vi "Set External Result Ref.vi"(10 "External Result Ref":string, 11 "Test Run Result in":refnum<class "Test Run Result.lvclass">) -> (3 "Test Run Result out":refnum<class "Test Run Result.lvclass">)   [LabVIEW 2026, in "Test Run Result.lvclass"]
uses:
  Test Run Result.lvclass
  Test Run Result.lvclass/Test Run Result.ctl
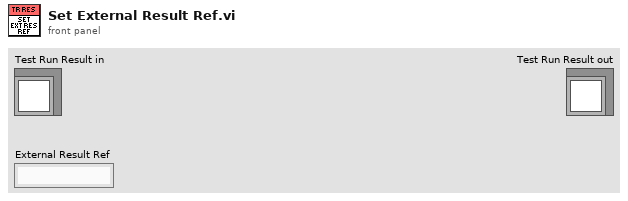
[diagram p1: front panel]
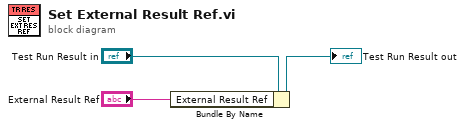
[diagram p0: block diagram]
diagram:
  n1 = Bundle By Name(cluster="Test Run Result in", "External Result Ref"="External Result Ref") -> (→"Test Run Result out":refnum<class "Test Run Result.lvclass">)
